vi "Unset Cursor Busy.vi"(8 "error in (no error)":errorcluster, 11 "UI in":refnum<class "UI.lvclass">) -> (0 "error out":errorcluster)   [LabVIEW 2020, in "AR Example.lvlib" / "UI.lvclass"]
uses:
  UI.lvclass
  UI.lvclass/UI.ctl
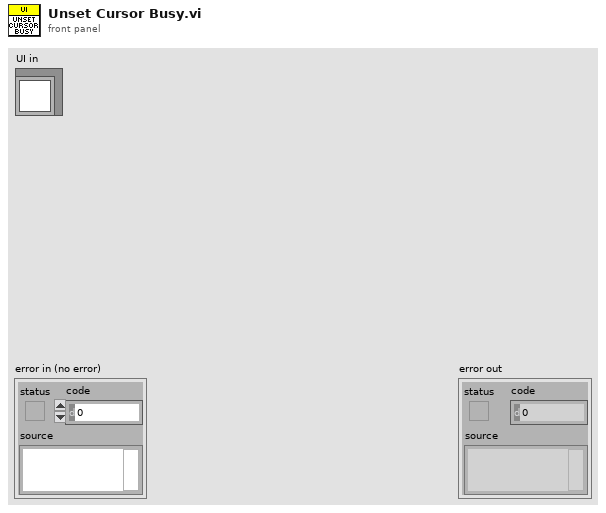
[diagram p1: front panel]
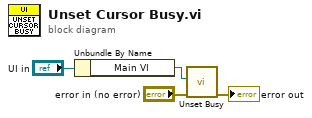
[diagram p0: block diagram]
diagram:
  n1 = Unbundle By Name("UI in") -> ("Main VI"=w3:refnum<vi>)
  n2 = call <vilib>:"Unset Busy.vi"("error in (no error)"="error in (no error)", "VI reference (current VI)"=w3) -> ("error out"=→"error out":errorcluster)  [unwired: 9 in]
